vi "my rio ir and cloud.vi"() -> ()   [LabVIEW 2015]
uses:
  <vilib>/httpClient/PUTBuffer.vi
  <vilib>/httpClient/LabVIEWHTTPClient.lvlib
panel:
  out "error out":errorcluster
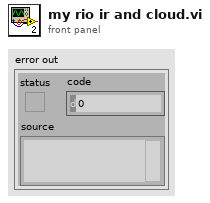
[diagram p1: front panel]
types:
  T1 = typedef "LabVIEWHTTPClient.lvlib/ClientHandle.ctl" = refnum<k1>
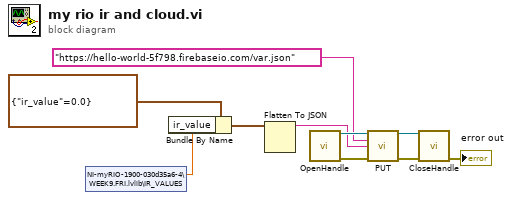
[diagram p0: block diagram]
diagram:
  n1 = shared-variable "NI-myRIO-1900-030d35a6-4\\WEEK9.FRI.lvlib\\IR_VALUES"() -> (w1:dbl)  [unwired: 1 in, 1 out]
  n2 = Bundle By Name(cluster=cluster{"ir_value":dbl} {"ir_value"=0.0}, "ir_value"=w1) -> (w3:cluster{"ir_value":dbl})
  n3 = Flatten To JSON(anything=w3) -> (JSON string=w4:string)  [unwired: 2 in, 1 out]
  n4 = call <vilib>:"OpenHandle.vi"() -> ("client handle out"=w10:T1, "error out"=w8:errorcluster)  [unwired: 14 in]
  n5 = call-poly <vilib>:"PUT.vi"("client handle"=w10, "url"="https://hello-world-5f798.firebaseio.com/var.json", "buffer"=w4, "error in (no error)"=w8) -> ("client handle out"=w9:T1, "error out"=w7:errorcluster)  [unwired: 8 in, 2 out]
  n6 = call <vilib>:"CloseHandle.vi"("client handle"=w9, "error in (no error)"=w7) -> ("error out"=→"error out":errorcluster)  [unwired: 13 in]
